vi "CLD 2  Elapsed Time Express with pause Self Solution.vi"() -> ()   [LabVIEW 2015]
doc: "CLD 2, Challenge Exercise"
panel:
  out "Elapsed Time (s)":dbl
  out "Time Has Elapsed":bool
  in  "Auto Reset":bool
  in  "Pause Button":bool
  in  "Reset Button":bool
  in  "Stop VI":bool
  out "error out":errorcluster
  in  "error in (no error)":errorcluster
  in  "Time Target (s)":dbl=7.0
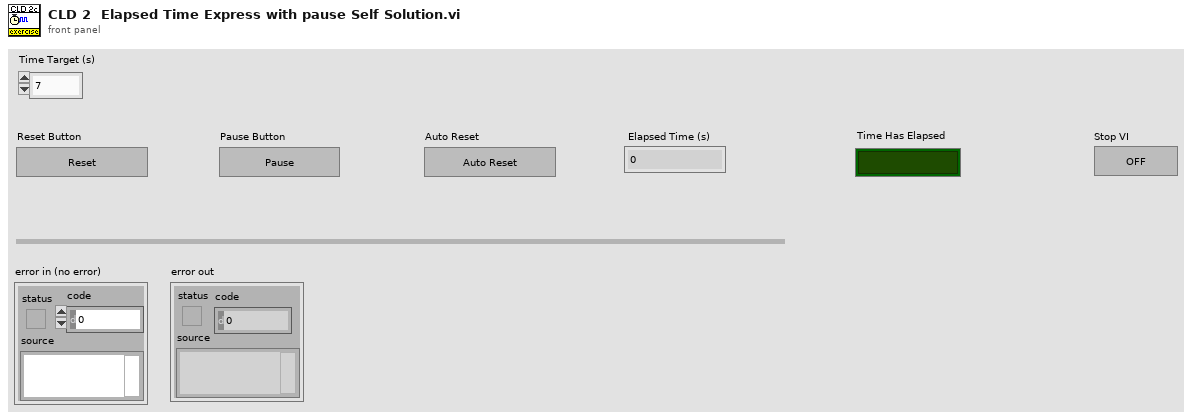
[diagram p1: front panel]
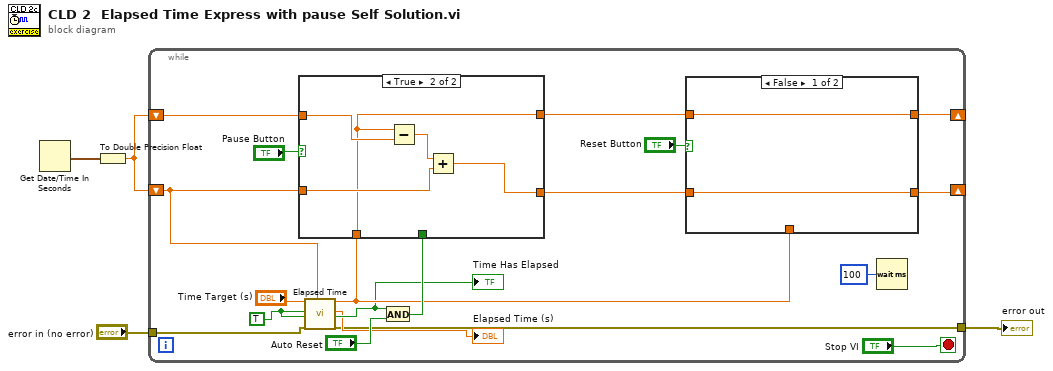
[diagram p0: block diagram]
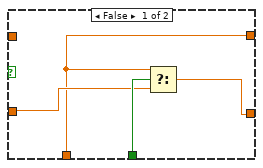
[diagram p3: hidden frame]
diagram:
  n1 = Get Date/Time In Seconds() -> (seconds since 1Jan1904=w4:timestamp)
  n2 = To Double Precision Float(number=w4) -> (double precision float=w3:dbl)
  n3 = while {
    shift-right: [w17] -> _
    shift-left: w3 -> [w21]
    shift-right: [w15] -> _
    shift-left: w3 -> [w20]
    tunnel: "error in (no error)" -> [w8]
    tunnel: [w7] -> w1
    stop <- "Stop VI" stop-if-true
    w6 = TRUE
    n4 = call "Elapsed Time"("Time Target (s)"="Time Target (s)", "Reset"=w6, "Auto Reset"=w6, "error in (no error)"=w8, "Set Start Time (s)"=w20) -> ("Present (s)"=w12:dbl, "Elapsed Time (s)"=→"Elapsed Time (s)":dbl, "Time has Elapsed"=w11:bool, "error out"=w7:errorcluster)  [unwired: 7 in, 4 out]
    "Time Has Elapsed" <- w11
    n5 = And(x=w11, y="Auto Reset") -> (x .and. y?=w13:bool)
    n6 = case shown="True" "Pause Button" {
      tunnel: w12 -> [w27 w32]
      tunnel: w21 -> [_ w35]
      tunnel: w20 -> [w29 w33]
      tunnel: [w27 w32] -> w18
      tunnel: [w28 w31] -> w16
      tunnel: w13 -> [w30 _]
      frame False {
        n7 = Select(t=w27, s=w30, f=w29) -> (s? t:f=w28:dbl)
      }
      frame True {
        n8 = Subtract(x=w32, y=w35) -> (x-y=w34:dbl)
        n9 = Add(x=w34, y=w33) -> (x+y=w31:dbl)
      }
    }
    n10 = case shown="False" "Reset Button" {
      tunnel: w18 -> [w25 _]
      tunnel: [w25 w26] -> w17
      tunnel: w16 -> [w24 _]
      tunnel: [w24 w26] -> w15
      tunnel: w12 -> [_ w26]
      frame False {
      }
      frame True {
      }
    }
    n11 = Wait (ms)(milliseconds to wait=u32 100) -> ()  [unwired: 1 out]
  }
  "error out" <- w1
